vi "InitialHeading.vi"() -> ()   [LabVIEW 2019]
panel:
  in  "Initial Heading":dbl
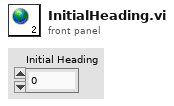
[diagram p1: front panel]
diagram:
